vi "nominal video create commit.vi"(8 "error in (no error)":errorcluster, 9 "out_video":i32, 10 "staging":i32, 11 "client":i32) -> (0 "error out":errorcluster, 1 "out_video out":i32, 3 "function return":i32)   [LabVIEW 2020, in "client.lvlib"]
doc: "int32_t nominal_video_create_commit(int32_t client, int32_t staging, int32_t *out_video);"
uses:
  client.lvlib
  nominalClient_64.dll
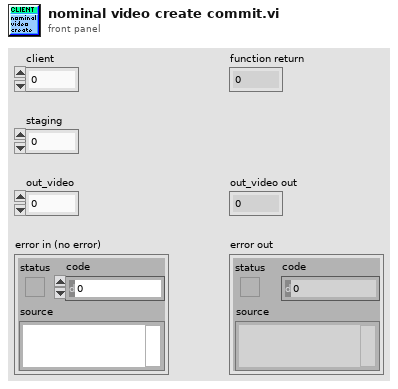
[diagram p1: front panel]
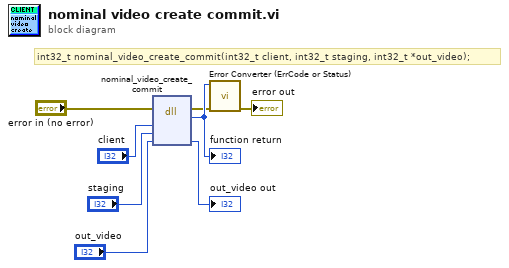
[diagram p0: block diagram]
diagram:
  # "int32_t nominal_video_create_commit(int32_t client, int32_t staging, int32_t *out_video);"
  n1 = dll-call lib="C:/code/labview-client-rs/lv_src/client/nominalClient_*.*" fn="nominal_video_create_commit"(error in="error in (no error)", "client"="client", "staging"="staging", "out_video"="out_video") -> (error out=w2:errorcluster, w8:i32, "out_video"=→"out_video out":i32)  [unwired: 4 in, 1 out]
  "function return" <- w8
  n2 = call "Error Converter (ErrCode or Status).vi"("error in (no error)"=w2, "error code"=w8) -> ("error out"=→"error out":errorcluster)  [unwired: 9 in]
